vi "SCLN_InitOldClient.vi"(2 "error in (no error)":errorcluster, 4 "Config File Name":path, 5 "Server  Name":string) -> (0 "error out":errorcluster, 1 "Add connection ID":refnum<k5>)   [LabVIEW 2015]
uses:
  SCLN_RW_Select.ctl
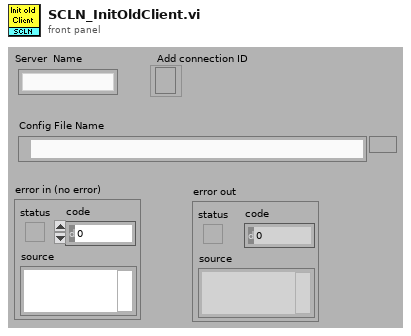
[diagram p1: front panel]
types:
  T1 = typedef "SCLN_InfoClusterConfig.ctl" = cluster{"Section Name":string, "IP_Server":string, "IP_Client":string, "IP_Port":string}
  T2 = typedef "SCLN_RW_Select.ctl" = enum16{"Read", "Write"}
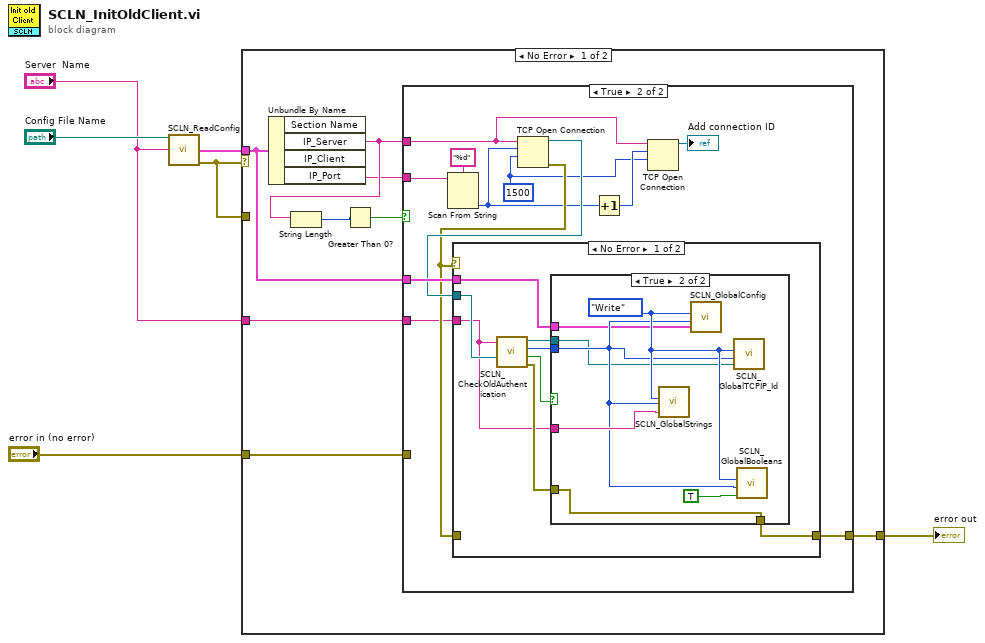
[diagram p0: block diagram]
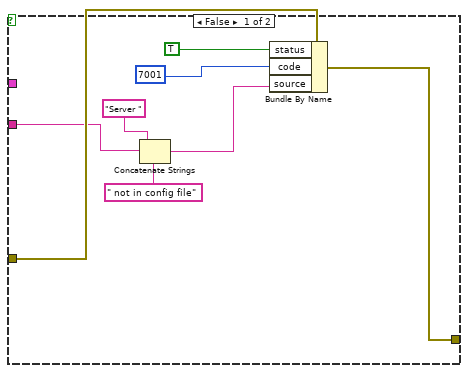
[diagram p2: hidden frame]
diagram:
  n1 = call "SCLN_ReadConfig.vi"("File Path"="Config File Name", "Section Name"="Server  Name") -> ("IP Info Connection"=w4:T1, "error out"=w3:errorcluster)  [unwired: 12 in]
  n2 = case shown="No Error" w3 {
    tunnel: w4 -> [w10 _]
    tunnel: [w9 w52] -> w2
    tunnel: "error in (no error)" -> [w8 _]
    tunnel: w3 -> [_ w52]
    tunnel: "Server  Name" -> [w7 _]
    frame No Error {
      n3 = Unbundle By Name(w10) -> ("IP_Server"=w12:string, "IP_Port"=w11:string)  [unwired: 2 out]
      n4 = String Length(string=w12) -> (length=w14:i32)
      n5 = Greater Than 0?(x=w14) -> (x > 0?=w13:bool)
      n6 = case shown="True" w13 {
        tunnel: w12 -> [_ w24]
        tunnel: w11 -> [_ w33]
        tunnel: w10 -> [_ w32]
        tunnel: [w16 w29] -> w9
        tunnel: w8 -> [w17 _]
        tunnel: w7 -> [w15 w28]
        frame False {
          n7 = Concatenate Strings("Server ", w15, " not in config file") -> (w18:string)
          n8 = Bundle By Name(cluster=w17, "status"=TRUE, "code"=7001, "source"=w18) -> (w16:errorcluster)
        }
        frame True {
          w25 = 1500
          n9 = Scan From String(format string="%d", input string=w33) -> (output 1=w27:i32)  [unwired: 3 in, 3 out]
          n10 = TCP Open Connection(address=w24, remote port or service name=w27, timeout ms (60000)=w25) -> (connection ID=w31:refnum<k5>, error out=w30:errorcluster)  [unwired: 2 in]
          n11 = case shown="No Error" w30 {
            tunnel: w32 -> [w36 _]
            tunnel: w31 -> [w42 _]
            tunnel: w30 -> [_ w51]
            tunnel: [w35 w51] -> w29
            tunnel: w28 -> [w37 _]
            frame No Error {
              n12 = call "SCLN_CheckOldAuthentication.vi"("Server Name"=w37, "TCP IN"=w42) -> ("TCP OUT"=w38:refnum<k5>, "Client Index"=w39:i32, "Authentic"=w41:bool, "error out"=w40:errorcluster)
              n13 = case shown="True" w41 {
                tunnel: w40 -> [w43 w44]
                tunnel: w39 -> [_ w47]
                tunnel: w38 -> [_ w46]
                tunnel: w37 -> [_ w48]
                tunnel: w36 -> [_ w45]
                tunnel: [w43 w44] -> w35
                frame False {
                }
                frame True {
                  w50 = SCLN_RW_Select."Write" ("GBL_RW")
                  n14 = call "SCLN_GlobalStrings.vi"("Write Value"=w48, "Element"=w47, "Operation"=w50) -> ()  [unwired: 1 in, 2 out]
                  n15 = call "SCLN_GlobalConfig.vi"("Write Value"=w45, "Element"=w47, "Operation"=w50) -> ()  [unwired: 1 in, 2 out]
                  n16 = call "SCLN_GlobalTCPIP_Id.vi"("TCPIP_Id Write"=w46, "Element"=w47, "Operation"=w50) -> ()  [unwired: 1 in, 2 out]
                  n17 = call "SCLN_GlobalBooleans.vi"("Write Value"=TRUE, "Element"=w47, "Operation"=w50) -> ()  [unwired: 1 in, 2 out]
                }
              }
            }
            frame Error {
            }
          }
          n18 = Increment(x=w27) -> (x+1=w26:i32)
          n19 = TCP Open Connection(address=w24, remote port or service name=w26, timeout ms (60000)=w25) -> (connection ID=→"Add connection ID":refnum<k5>)  [unwired: 2 in, 1 out]
        }
      }
    }
    frame Error {
    }
  }
  "error out" <- w2
